vi "Switch Configure (Poly).vi"   [LabVIEW 2016, in "Hall Effect Library.lvlib"]
uses:
  Hall Effect Library.lvlib
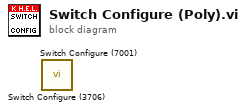
[diagram p0: block diagram]
diagram:
  n1 = call "Switch Configure (3706).vi"() -> ()  [unwired: 10 in, 2 out]
  n2 = call "Switch Configure (7001).vi"() -> ()  [unwired: 10 in, 2 out]
